vi "Datalogger Headers Set Message Create.vi"(8 "error in (no error)":errorcluster, 10 "Headers":string[](array[string]), 11 "Datalogger Headers Set Message in":refnum<class "Datalogger Headers Set Message.lvclass">) -> (0 "error out":errorcluster, 3 "Datalogger Headers Set Message out":refnum<class "Datalogger Headers Set Message.lvclass">)   [LabVIEW 2018, in "Datalogger Headers Set Message.lvclass"]
uses:
  Datalogger Headers Set Message.lvclass
  Datalogger Headers Set Message.lvclass/Datalogger Headers Set Message.ctl
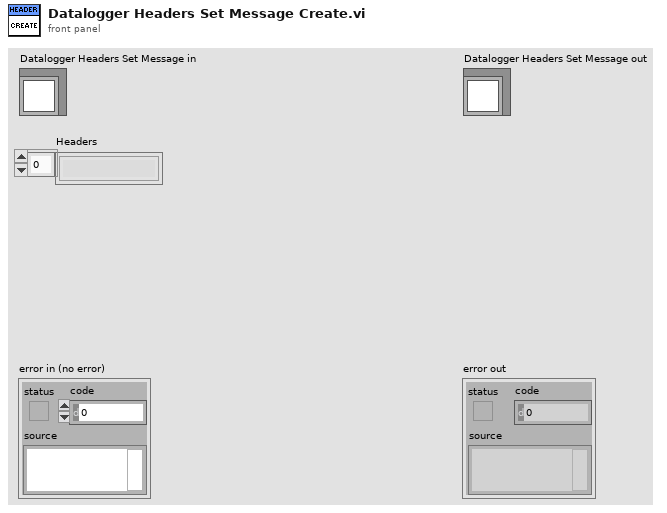
[diagram p1: front panel]
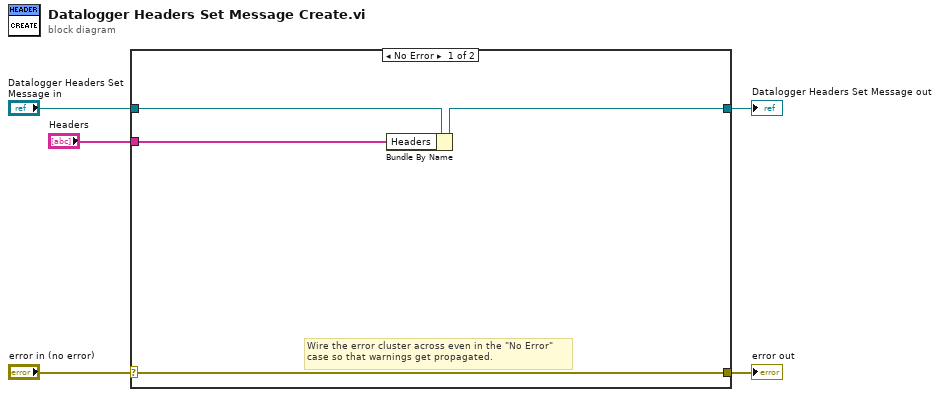
[diagram p0: block diagram]
diagram:
  n1 = case shown="No Error" "error in (no error)" {
    selector: "error in (no error)" -> [w9 w11]
    tunnel: [w9 w11] -> w4
    tunnel: [w6 w10] -> w2
    tunnel: "Datalogger Headers Set Message in" -> [w8 w10]
    tunnel: "Headers" -> [w7 _]
    frame No Error {
      # "Wire the error cluster across even in the \"No Error\"\ncase so that warnings get propagated."
      n2 = Bundle By Name(cluster=w8, "Headers"=w7) -> (w6:refnum<class "Datalogger Headers Set Message.lvclass">)
    }
    frame Error {
    }
  }
  "error out" <- w4
  "Datalogger Headers Set Message out" <- w2
